vi "compute_point_sweep.vi"(8 "steps":u16, 9 "index":u16, 10 "call type":T2, 11 "mag field":T1) -> (1 "New value":sgl, 2 "mag fiel parms out":T1)   [LabVIEW 2010]
uses:
  type defs - instruments/usage.ctl
  type defs - instruments/sweep info.ctl
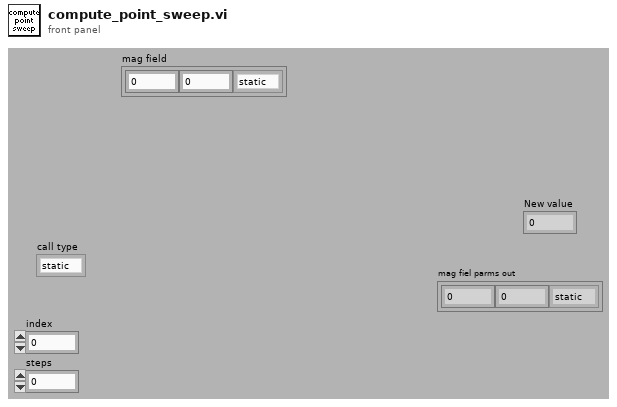
[diagram p1: front panel]
types:
  T1 = typedef "sweep info.ctl" = cluster{"from":sgl, "to":sgl, "type":T2}
  T2 = typedef "usage.ctl" = enum8{"static", "sweep", "step", "step 2", "step 3"}
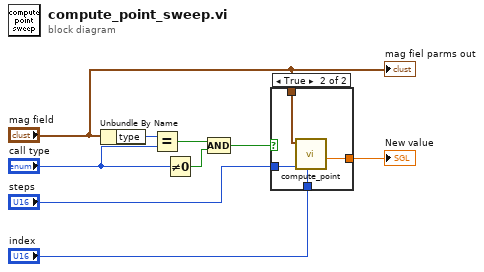
[diagram p0: block diagram]
diagram:
  n1 = Unbundle By Name("mag field") -> ("type"=w7:T2)
  n2 = Equal?(x=w7, y="call type") -> (x = y?=w6:bool)
  n3 = Not Equal To 0?(x="call type") -> (x != 0?=w5:bool)
  n4 = Compound Arithmetic op=AND(w6, w5) -> (w4:bool)
  n5 = case shown="True" w4 {
    tunnel: "mag field" -> [_ w10]
    tunnel: "index" -> [_ w13]
    tunnel: "steps" -> [_ w12]
    tunnel: [_ w11] -> w2
    frame False {
    }
    frame True {
      n6 = call "compute_point.vi"("sweep index"=w13, "steps"=w12, "sweep infos"=w10) -> ("Numeric"=w11:sgl)  [unwired: 1 in, 7 out]
    }
  }
  "New value" <- w2
  "mag fiel parms out" <- "mag field"
